vi "Get Time64.vi"() -> (0 "Labview time (ms)":u64)   [LabVIEW 2009, in "Time.lvlib"]
uses:
  Time.lvlib
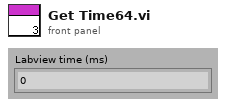
[diagram p1: front panel]
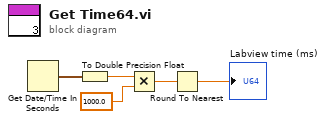
[diagram p0: block diagram]
diagram:
  n1 = Get Date/Time In Seconds() -> (seconds since 1Jan1904=w5:timestamp)
  n2 = To Double Precision Float(number=w5) -> (double precision float=w1:dbl)
  n3 = Multiply(x=w1, y=1000.0) -> (x*y=w3:dbl)
  n4 = Round To Nearest(number=w3) -> (nearest integer value=→"Labview time (ms)":dbl)
